vi "DO calibrator.vi"(7 "Scales in":T7 {"D.O."."K" format="%.6f"; "D.O."."Temperature" format="%.2f"; "pH scale"."Buffers"."V/T" format="%.5f"; "pH scale"."Buffers"."Buffer" format="%.2f"; "pH scale"."Temperature" format="%.2f"; "offset (physical units)" format="%.5f"; "correspondence table"."volts" format="%.4f"; "correspondence table"."physical units" format="%.4f"; "second channel" min=-1; "offset (volts)" format="%.5f"; "conversion matrix" format="%.4e"}, 8 "Server Stats":T8={"scan rate"=10.0, "# connections"=0, "channel settings"=[]} {"channel settings"."lower input limits" format="%.4f"; "channel settings"."upper input limits" format="%.4f"; "scan rate" format="%.2f"}, 9 "method":T9={"sampling interval"=0.1, "samples to average"=1, "data interval"=0.0, "stream data"=FALSE, "file path"=refnum, "command"={"command"=enum."Idle", "start time (ms)"=0, "Channel Indices"=[], "Scans per Sample"=1}} {"command"."Scans per Sample" min=1; "data interval" format="%.2f"; "samples to average" min=1 step=1; "sampling interval" format="%.2f"}, 10 "channel index":i8, 11 "Connection ID":refnum<k5>) -> (3 "Scaling":T1={"conversion matrix"=[[0.0, 0.0], [0.0, 0.0], [0.0, 0.0], [0.0, 0.0], [0.0, 0.0], [0.0, 0.0]], "units"="", "name"="", "scale type"=enum."Volts", "offset (volts)"=0.0, "second channel"=0, "correspondence table"=[], "offset (physical units)"=0.0, "pH scale"={"Buffers"=[], "Temperature"=0.0}, "D.O."={"Temperature"=0.0, "K"=0.0, "barometric pressure"=0.0}} {"D.O."."K" format="%.6f"; "D.O."."Temperature" format="%.2f"; "pH scale"."Buffers"."V/T" format="%.5f"; "pH scale"."Buffers"."Buffer" format="%.2f"; "pH scale"."Temperature" format="%.2f"; "offset (physical units)" format="%.5f"; "correspondence table"."volts" format="%.4f"; "correspondence table"."physical units" format="%.4f"; "second channel" min=-1; "offset (volts)" format="%.5f"; "conversion matrix" format="%.4e"})   [LabVIEW 2010]
doc: "Illustrates the simplest form of TCP data acquisition using a TCP data server.\n\n\nCreated by Monroe Weber-Shirk\nCornell University\nmw24@cornell.edu\nJanuary 2000"
uses:
  <vilib>/Analysis/NI_AALBase.lvlib
  DataServer/command.ctl
  DataServer/command cluster.ctl
  DAC apps/support/method.ctl
  DataServer/Server stats.ctl
  conversion.ctl
  correspondence table.ctl
  DAQ configuration/scale type.ctl
  calib array.ctl
  pH/pH scale.ctl
  DO scale.ctl
panel:
  in  "OK Button":bool
  in  "Tab Control":enum32{"Calibrate", "Help"}(tab)
  out "Temperature compensated":bool
  out "DO sat (mg/L)":dbl format="%.2f"
  in  "Barometric Pressure (kPa)":dbl=101.3 format="%.2f"
  in  "Temperature (C)":dbl=20.0 format="%.2f"
  out "sample time":dbl format="%.2f"
  out "Sample rate":dbl format="%.2f"
  in  "data points to acquire":u32=1000 min=1
  in  "Scans per Sample":i32=1 min=1
  in  "command state":T6
  # "Hz"
  # "s"
  # "C"
  # "kPa"
  # "C"
  # "Enter the barometric pressure. If you are not using a second channel for temperature compensation, then enter the sample temperature.\nEnter an appropriate sample time by changing the data points to acquire (10 seconds of sampling is reasonable).\n\nPlace the probe in moist air or saturated water (saturated water seems to work best).\nSelect \"Measure Saturation\" from the control palette. The voltage reading should be between 0.18 V and 0.20 V if the membrane is in good condition and the air temperature is between 20 and 25C.\n\nIf desired you can save the calibration to file for later use. The calibration will be available for Signal Monitor to use now even if you don't save the file.\n\nIf the sample temperature or barometric pressure changes you can return to this dialog box to change them. It isn't necessary to rerun the calibration! Correct sample temperature is important because the oxygen diffusion rate increases with temperature. If possible use a temperature probe and link the temperature probe to the DO probe by selecting it as a second channel."
  # "C"
  # "kPa"
  # "C"
  # "Hz"
  # "s"
  # "s"
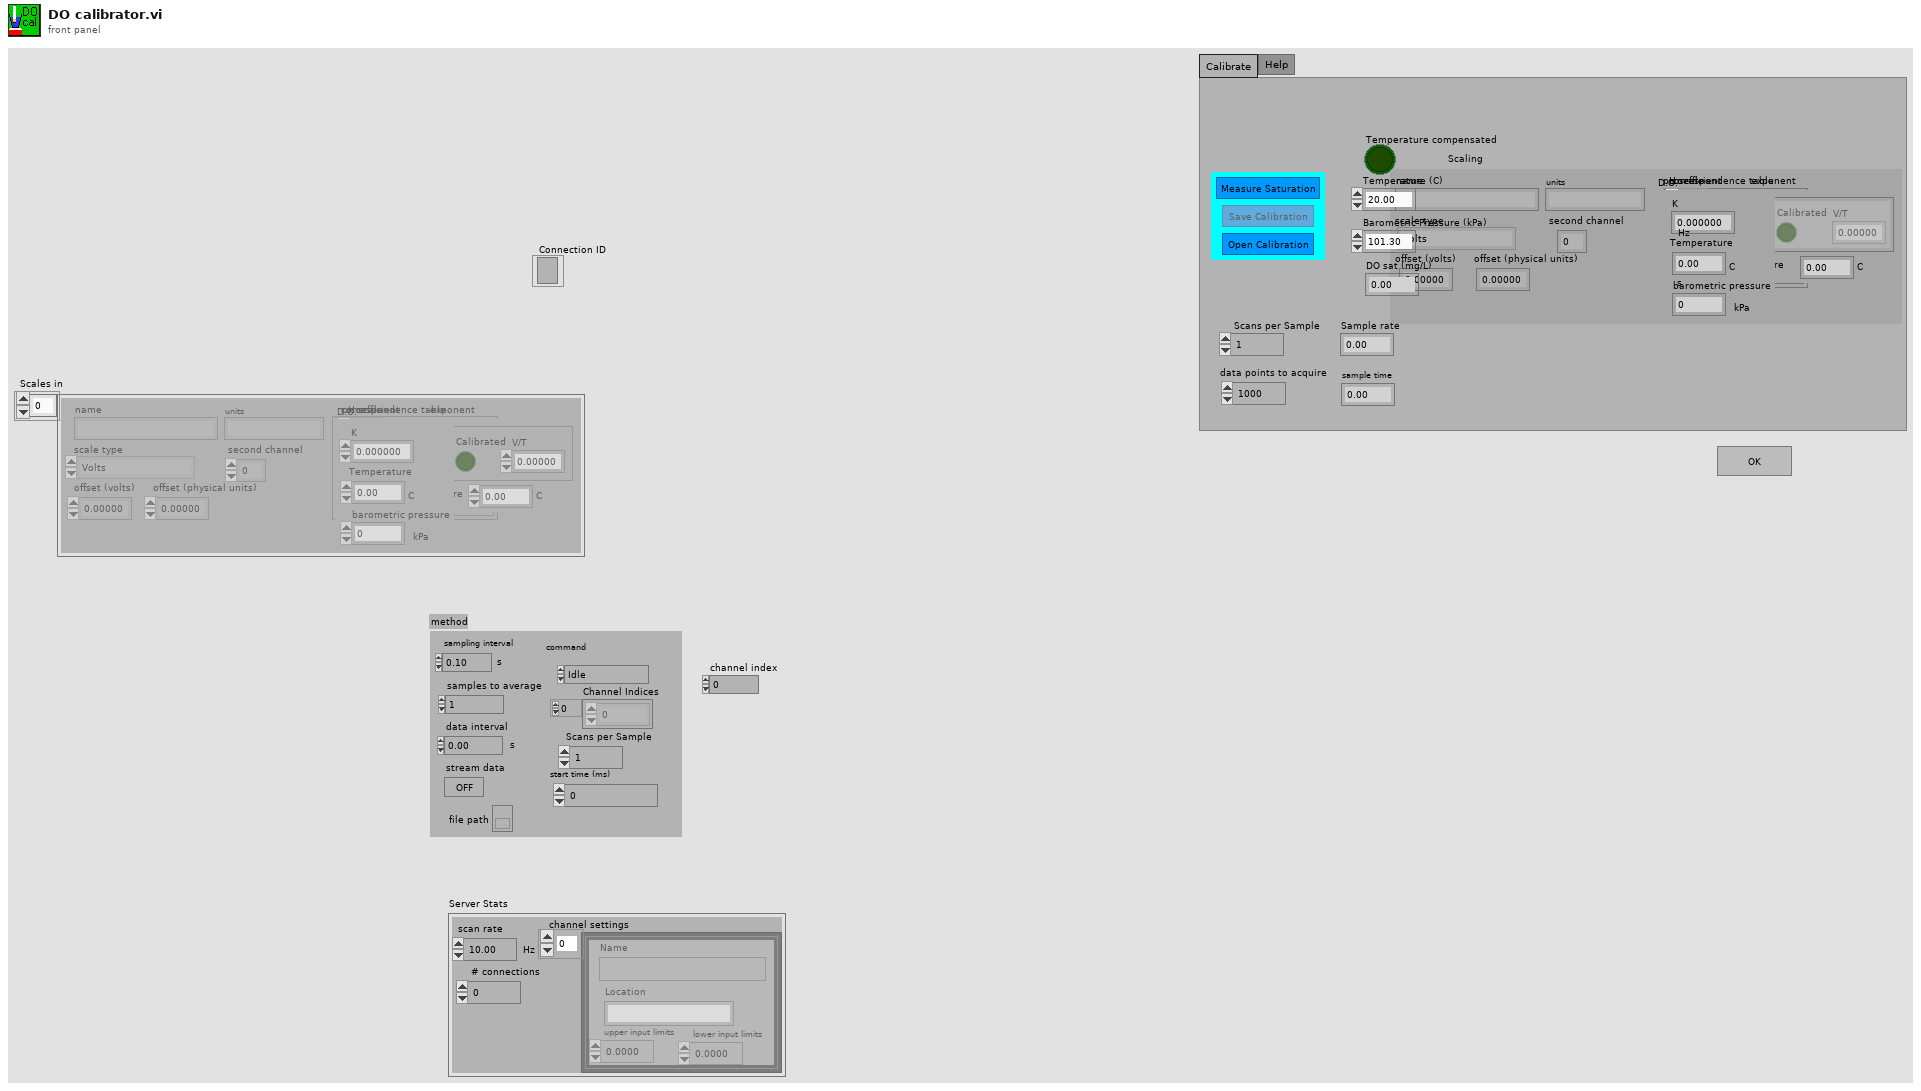
[diagram p1: front panel]
types:
  T1 = typedef "conversion.ctl" = cluster{"conversion matrix":sgl[][], "units":string, "name":string, "scale type":T2, "offset (volts)":dbl, "second channel":i8, "correspondence table":T3, "offset (physical units)":dbl, "pH scale":T4, "D.O.":T5}
  T2 = typedef "scale type.ctl" = enum16{"Volts", "Polynomial", "Correspondence Table", "pH", "Dissolved Oxygen", "Quadratic"}
  T3 = typedef "correspondence table.ctl" = cluster{"physical units":dbl, "volts":dbl}[]
  T4 = typedef "pH scale.ctl" = cluster{"Buffers":cluster{"Buffer":dbl, "Calibrated":bool, "V/T":dbl}[], "Temperature":dbl}
  T5 = typedef "DO scale.ctl" = cluster{"Temperature":dbl, "K":dbl, "barometric pressure":dbl}
  T6 = cluster{"Measure Saturation":bool, "Save Calibration":bool, "Save Calibration 2":bool}
  T7 = typedef "calib array.ctl" = T1[]
  T8 = typedef "Server stats.ctl" = cluster{"scan rate":dbl, "# connections":i32, "channel settings":cluster{"Name":string, "upper input limits":sgl, "lower input limits":sgl, "Location":string}[]}
  T9 = typedef "method.ctl" = cluster{"sampling interval":sgl, "samples to average":u32, "data interval":sgl, "stream data":bool, "file path":refnum<file>, "command":T10}
  T10 = typedef "command cluster.ctl" = cluster{"command":T11, "start time (ms)":u32, "Channel Indices":i32[], "Scans per Sample":i32}
  T11 = typedef "command.ctl" = enum16{"Idle", "Send Data", "Send 1 Scan", "Logoff"}
  T12 = enum16{"Volts", "Polynomial", "Correspondence Table", "pH", "Dissolved Oxygen"}
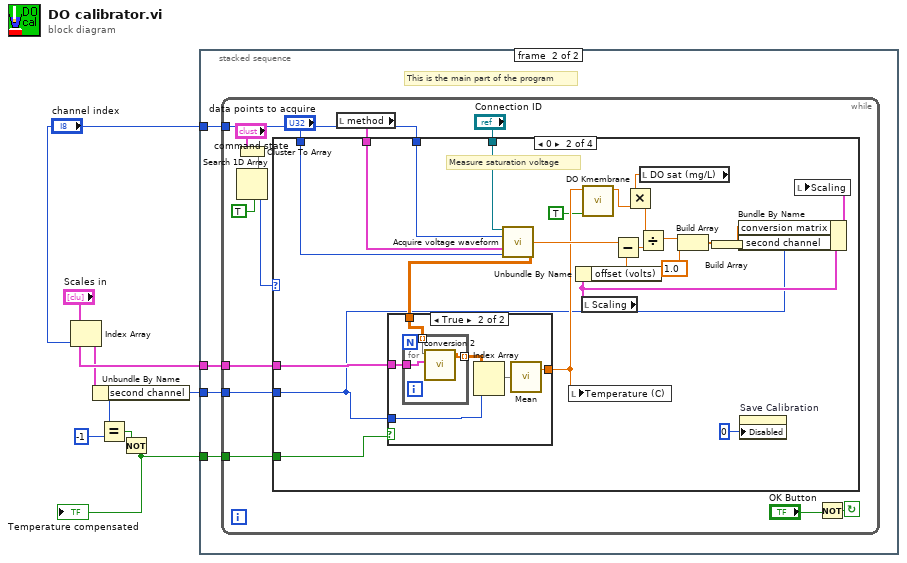
[diagram p0: block diagram]
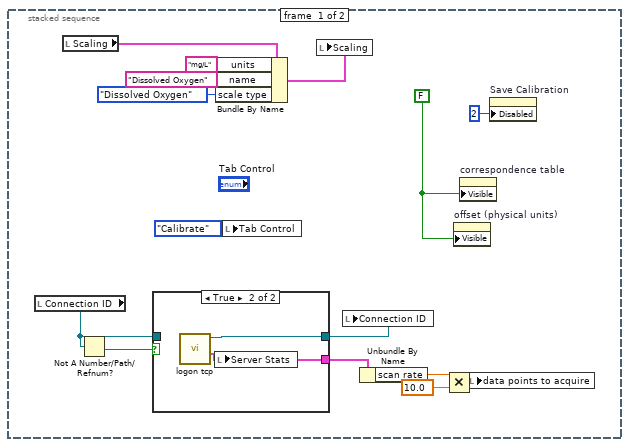
[diagram p2: hidden frame]
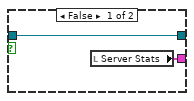
[diagram p3: hidden frame]
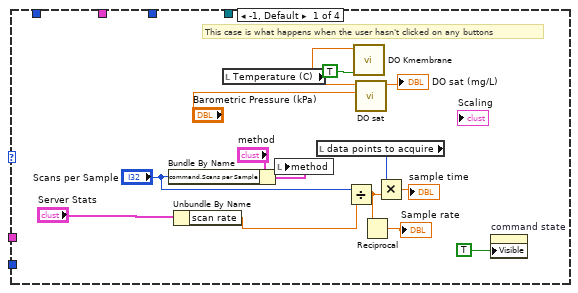
[diagram p4: hidden frame]
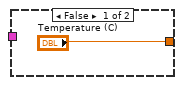
[diagram p5: hidden frame]
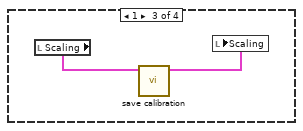
[diagram p6: hidden frame]
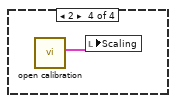
[diagram p7: hidden frame]
diagram:
  n1 = Index Array(array="Scales in", index="channel index") -> (element=w5:T1)
  n2 = Unbundle By Name(w5) -> ("second channel"=w4:i8)
  n3 = Equal?(x=w4, y=i8 -1) -> (x = y?=w2:bool)
  n4 = Not(x=w2) -> (.not. x?=w1:bool)
  "Temperature compensated" <- w1
  n5 = stacked-sequence {
    tunnel: "channel index" -> [_ w30]
    tunnel: w4 -> [_ w29]
    tunnel: w1 -> [_ w28]
    tunnel: "Scales in" -> [_ w27]
    frame #0 {
      w9 = FALSE ("Visible")
      n6 = local read "Connection ID"() -> (w20:refnum<k5>)
      n7 = local read "Scaling"() -> (w19:T1)
      n8 = Not A Number/Path/Refnum?(number/path/refnum=w20) -> (NaN/Path/Refnum?=w22:bool)
      n9 = case shown="True" w22 {
        tunnel: [w24 w26] -> w21
        tunnel: w20 -> [w24 _]
        tunnel: [w23 w25] -> w14
        frame False {
          n10 = local read "Server Stats"() -> (w23:T8)
        }
        frame True {
          n11 = call "logon tcp.vi"() -> ("Server stats"=w25:T8, "connection ID"=w26:refnum<k5>)  [unwired: 6 in, 4 out]
          n12 = local write "Server Stats"(w25) -> ()
        }
      }
      n13 = Bundle By Name(cluster=w19, "units"="mg/L", "name"="Dissolved Oxygen", "scale type"=T12."Dissolved Oxygen") -> (w18:T1)
      n14 = local write "Tab Control"(enum32{"Calibrate", "Help"}."Calibrate" ("Tab Control")) -> ()
      n15 = local write "Scaling"(w18) -> ()
      n16 = local write "Connection ID"(w21) -> ()
      n17 = Unbundle By Name(w14) -> ("scan rate"=w13:dbl)
      n18 = Multiply(x=w13, y=10.0) -> (x*y=w11:dbl)
      n19 = property on="offset (physical units)" class="DigNum (strict)"("Visible"=w9) -> ()  [unwired: 2 in, 2 out]
      n20 = property on="correspondence table" class="Arr (strict)"("Visible"=w9) -> ()  [unwired: 2 in, 2 out]
      n21 = local write "data points to acquire"(w11) -> ()
      n22 = property on="Save Calibration" class="Bool"("Disabled"=u8 2) -> ()  [unwired: 2 in, 2 out]
    }
    frame #1 {
      # "This is the main part of the program"
      n23 = while {
        tunnel: w27 -> [w31]
        tunnel: w28 -> [w32]
        tunnel: w29 -> [w33]
        tunnel: w30 -> [w34]
        stop <- w43 continue-if-true
        n24 = Cluster To Array(cluster="command state") -> (array=w41:bool[])
        n25 = Search 1D Array(1D array=w41, element=TRUE) -> (index of element=w39:i32)  [unwired: 1 in]
        n26 = local read "method"() -> (w37:T9)
        n27 = case shown="0" w39 {
          tunnel: "Connection ID" -> [_ w80 _ _]
          tunnel: w34 -> [_ w64 _ _]
          tunnel: w37 -> [_ w79 _ _]
          tunnel: "data points to acquire" -> [_ w78 _ _]
          tunnel: w33 -> [_ w58 _ _]
          tunnel: w32 -> [_ w62 _ _]
          tunnel: w31 -> [_ w61 _ _]
          frame -1, Default {
            # "This case is what happens when the user hasn't clicked on any buttons"
            n28 = Bundle By Name(cluster="method", "command.Scans per Sample"="Scans per Sample") -> (w53:T9)
            n29 = Unbundle By Name("Server Stats") -> ("scan rate"=w56:dbl)
            n30 = local read "Temperature (C)"() -> (w45:dbl)
            n31 = local write "method"(w53) -> ()
            n32 = local read "data points to acquire"() -> (w51:u32)
            n33 = Divide(x="Scans per Sample", y=w56) -> (x/y=w49:dbl)
            n34 = call "DO Kmembrane.vi"(8:TRUE ("initialize Temperature"), "Temperature (C)"=w45) -> ()  [unwired: 9 in, 1 out]
            n35 = call "DO sat.vi"("Atmospheric Pressure (kPa)"="Barometric Pressure (kPa)", "Temperature (C)"=w45) -> ("DO sat (mg/L)"=→"DO sat (mg/L)":dbl)  [unwired: 9 in]
            n36 = Reciprocal(x=w49) -> (1/x=→"Sample rate":dbl)
            n37 = Multiply(x=w51, y=w49) -> (x*y=→"sample time":dbl)
            n38 = property on="command state" class="Clust"("Visible"=TRUE ("Write Attribute")) -> ()  [unwired: 2 in, 2 out]
          }
          frame 0 {
            # "Measure saturation voltage"
            n39 = call "Acquire voltage waveform.vi"("Connection ID"=w80, "channel index"=w64, "method"=w79, "data points to acquire"=w78) -> ("mean"=w76:dbl, "all data"=w65:sgl[][])  [unwired: 6 in, 4 out]
            n40 = case shown="True" w62 {
              tunnel: w65 -> [_ w87]
              tunnel: w61 -> [_ w84]
              tunnel: w58 -> [_ w83]
              tunnel: ["Temperature (C)" w82] -> w63
              frame False {
              }
              frame True {
                n41 = for {
                  tunnel: w84 -> [w90]
                  tunnel: w87 -> [w89] mode=indexing
                  tunnel: [w88] -> w86 mode=indexing
                  n42 = call "conversion 2.vi"(10:w90, "voltage data"=w89) -> ("calibrated data"=w88:sgl[])  [unwired: 8 in, 1 out]
                }
                n43 = Index Array(array=w86, index (col)=w83) -> (element=w85:sgl[])  [unwired: 1 in]
                n44 = call <vilib>:"Mean.vi"("X"=w85) -> ("mean"=w82:dbl)  [unwired: 1 out]
              }
            }
            n45 = local write "Temperature (C)"(w63) -> ()
            n46 = local read "Scaling"() -> (w77:T1)
            n47 = Unbundle By Name(w77) -> ("offset (volts)"=w75:dbl)
            n48 = call "DO Kmembrane.vi"(8:TRUE ("initialize Temperature"), "Temperature (C)"=w63) -> ("Kmembrane"=w68:dbl)  [unwired: 9 in]
            n49 = Subtract(x=w76, y=w75) -> (x-y=w74:dbl)
            n50 = local read "DO sat (mg/L)"() -> (w67:dbl)
            n51 = Multiply(x=w67, y=w68) -> (x*y=w66:dbl)
            n52 = Divide(x=w66, y=w74) -> (x/y=w71:dbl)
            n53 = Build Array(w71, 1.0 ("Input Element")) -> (w73:dbl[])
            n54 = Build Array(w73) -> (w72:dbl[][])
            n55 = Bundle By Name(cluster=w77, "conversion matrix"=w72, "second channel"=w58) -> (w69:T1)
            n56 = property on="Save Calibration" class="Bool"("Disabled"=u8 0) -> ()  [unwired: 2 in, 2 out]
            n57 = local write "Scaling"(w69) -> ()
          }
          frame 1 {
            n58 = local read "Scaling"() -> (w92:T1)
            n59 = call "save calibration.vi"("conversion in"=w92) -> ("conversion out"=w91:T1)  [unwired: 6 in]
            n60 = local write "Scaling"(w91) -> ()
          }
          frame 2 {
            n61 = call "open calibration.vi"() -> ("conversion out"=w93:T1)  [unwired: 7 in]
            n62 = local write "Scaling"(w93) -> ()
          }
        }
        n63 = Not(x="OK Button") -> (.not. x?=w43:bool)
      }
    }
  }
